vi "Main.vi"(11 "Module Admin":refnum<class "Delacor_lib_QMH_Module Admin.lvclass">) -> ()   [LabVIEW 2024, in "ControllerUI.lvlib"]
doc: "This template is based off of the Queued Message Handler design pattern and the Queued Message Handler project template that ships with LabVIEW.\n\nThe main difference is that the queue is private to this module and communication between modules is performed via Broadcast and Request events.\n\nRequest events are wrapped in public API methods and are handled in the Event Handling Loop (EHL) of this VI. Any module can register for Broadcast events sent by this module. The EHL generates messages based on user interface actions.\n\nThe Message Handling Loop (MHL) processes messages generated by the EHL, or by other messages. The messages are string values, so new messages can be added easily to the Message Cases case structure in the MHL. Each message cluster can also provide an optional value for Message Data, which is a variant that can be converted to whatever message-specific data is required.\n_____\nBased on DQMH Dev Tools: Project Template 7.1.0.1503."
uses:
  ControllerUI.lvlib
  <vilib>/Delacor/Delacor QMH/Libraries/Module Admin_class/Delacor_lib_QMH_Module Admin.lvclass
  Module Data--cluster.ctl
  <vilib>/Utility/miscctls.llb/LVFontTypeDef.ctl
  Stop Argument--cluster.ctl
  <vilib>/Delacor/Delacor QMH/Libraries/Message Queue_class/Delacor_lib_QMH_Message Queue.lvclass/Delacor_lib_QMH_Message Queue.ctl
  <vilib>/Delacor/Delacor QMH/Libraries/Module Admin_class/Delacor_lib_QMH_Module Admin.lvclass/Delacor_lib_QMH_Module Admin.ctl
  <vilib>/Delacor/Delacor QMH/Libraries/Message Queue_class/Delacor_lib_QMH_Enqueue Message (Single).vi
  <vilib>/Delacor/Delacor QMH/Libraries/Module Admin_class/Delacor_lib_QMH_Get External Launch.vi
  <vilib>/Delacor/Delacor QMH/Libraries/Message Queue_class/Delacor_lib_QMH_Message Queue.lvclass
  MoneyControl/MoneyControl.lvlib
  ProductControl/ProductControl.lvlib
  <vilib>/PantherLAB/Message Module/Libraries/Message/PantherLAB_lib_Message.lvlib
panel:
  out "error out":errorcluster
  out "Status":string
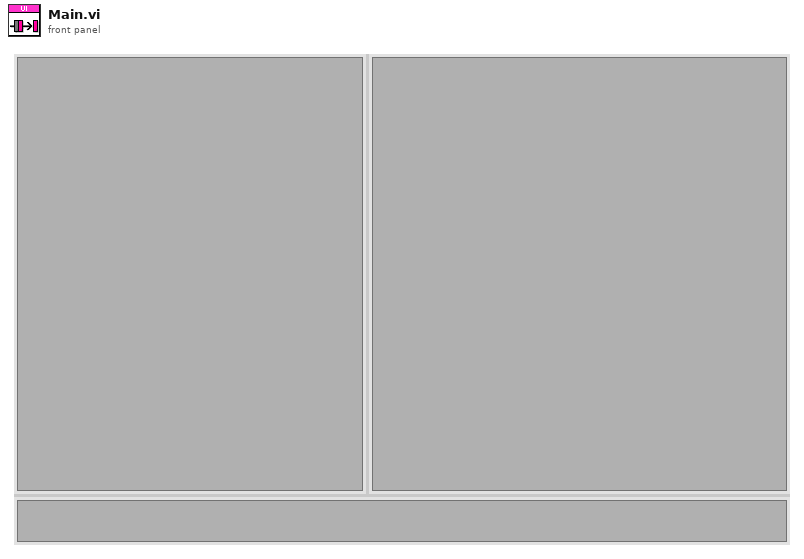
[diagram p1: front panel]
types:
  T1 = typedef "ControllerUI.lvlib/Request Events--cluster.ctl" = cluster{"Stop Module":refnum<user-event>, "Show Panel":refnum<user-event>, "Hide Panel":refnum<user-event>, "Get Module Execution Status":refnum<user-event>, "Show Diagram":refnum<user-event>}
  T2 = typedef "PantherLAB_lib_Message.lvlib/Broadcast Events--cluster.ctl" = cluster{"Module Did Init":refnum<user-event>, "Status Updated":refnum<user-event>, "Error Reported":refnum<user-event>, "Module Did Stop":refnum<user-event>, "Update Module Execution Status":refnum<user-event>}
  T3 = typedef "MoneyControl.lvlib/Broadcast Events--cluster.ctl" = cluster{"Module Did Init":refnum<user-event>, "Status Updated":refnum<user-event>, "Error Reported":refnum<user-event>, "Module Did Stop":refnum<user-event>, "Update Module Execution Status":refnum<user-event>, "Credito Actualizado":refnum<user-event>}
  T4 = typedef "ProductControl.lvlib/Broadcast Events--cluster.ctl" = cluster{"Module Did Init":refnum<user-event>, "Status Updated":refnum<user-event>, "Error Reported":refnum<user-event>, "Module Did Stop":refnum<user-event>, "Update Module Execution Status":refnum<user-event>, "Seleccion Producto Actualizada":refnum<user-event>}
  T5 = typedef "ControllerUI.lvlib/Module Data--cluster.ctl" = cluster{"Status":string}
  T6 = typedef "LVFontTypeDef.ctl" = cluster{"Font Name":string, "Size":u16, "Bold":bool, "Italic":bool, "Underline":bool, "Strikeout":bool, "Color":u32}
  T7 = enum32{"invalid lock state", "Not Locked", "Locked (No Password)", "Password-protected"}
  T8 = typedef "ControllerUI.lvlib/Stop Argument--cluster.ctl" = cluster{"Origin":string, "Exit via Stop Module Req?":bool, "Wait for Module to stop?":bool}
  T9 = enum32{"Invalid", "Standard", "Closed", "Hidden", "Minimized", "Maximized"}
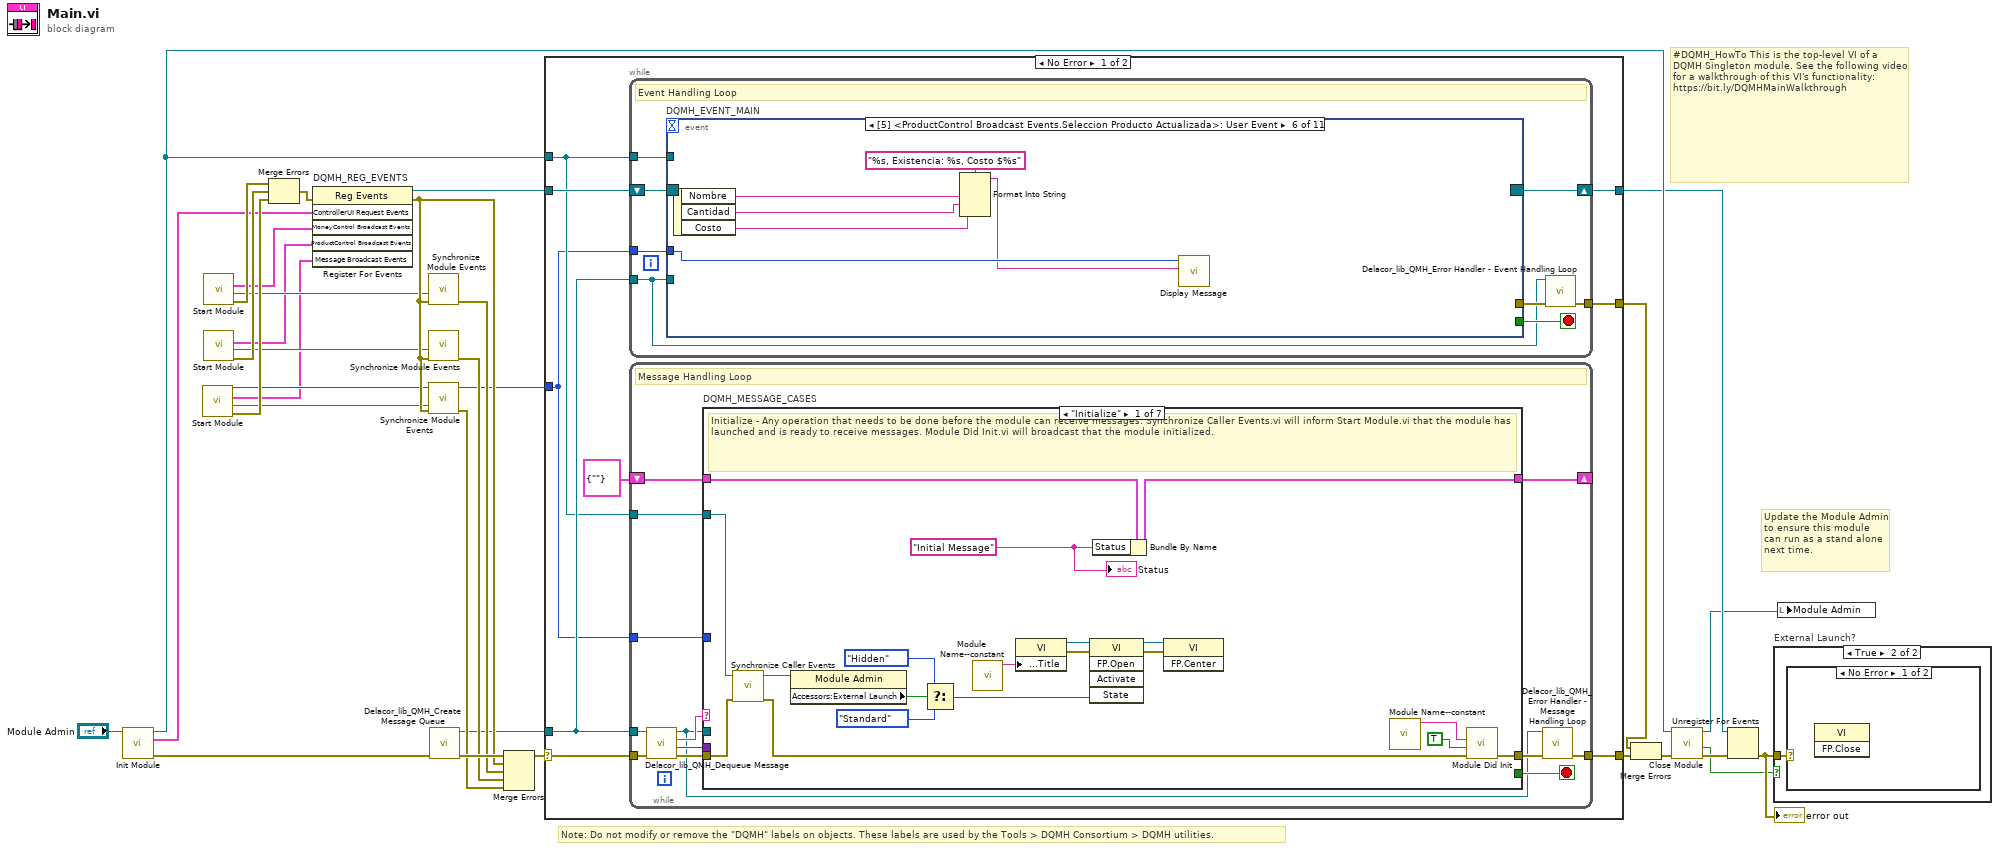
[diagram p0: block diagram]
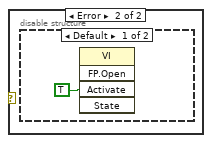
[diagram p3: hidden frame]
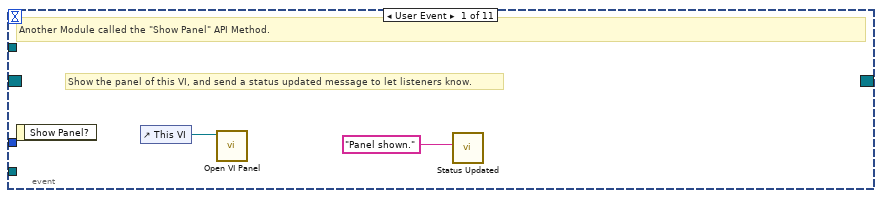
[diagram p5: hidden frame]
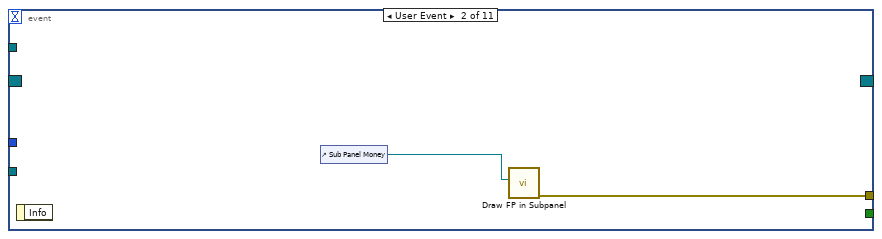
[diagram p6: hidden frame]
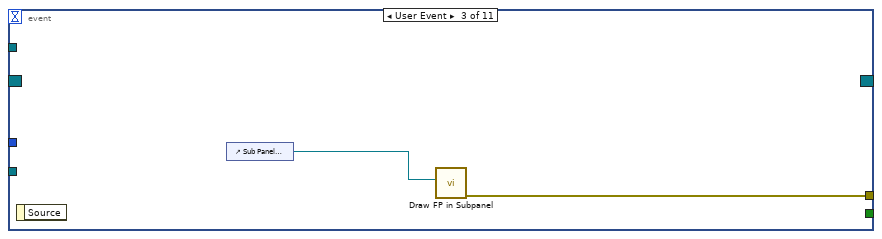
[diagram p7: hidden frame]
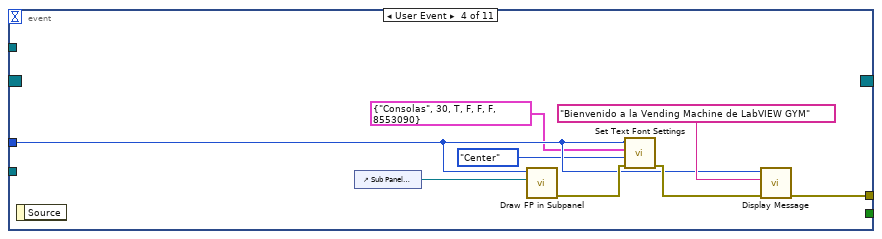
[diagram p8: hidden frame]
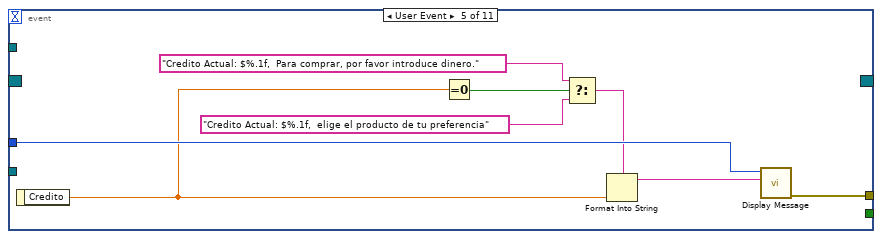
[diagram p9: hidden frame]
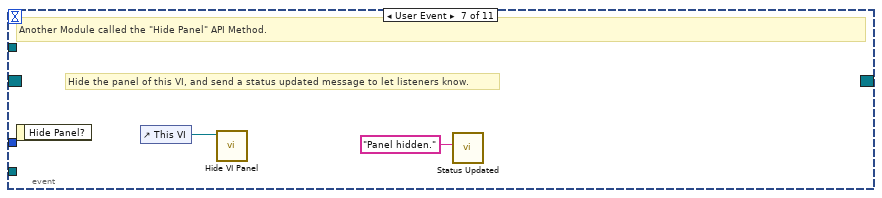
[diagram p10: hidden frame]
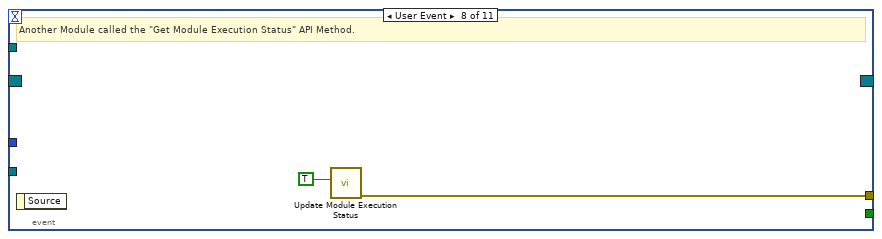
[diagram p11: hidden frame]
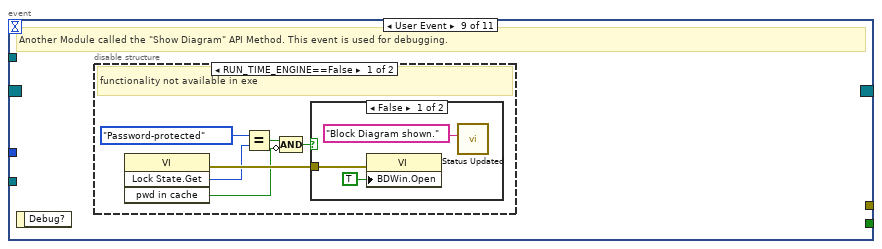
[diagram p12: hidden frame]
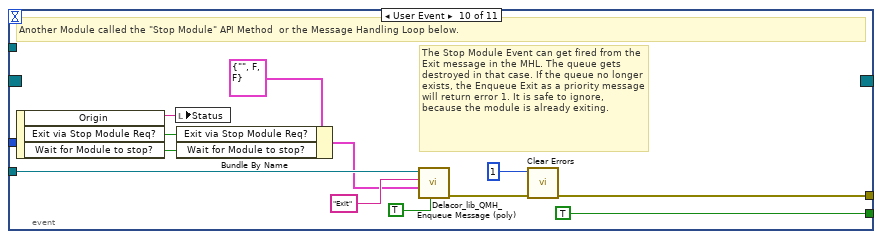
[diagram p15: hidden frame]
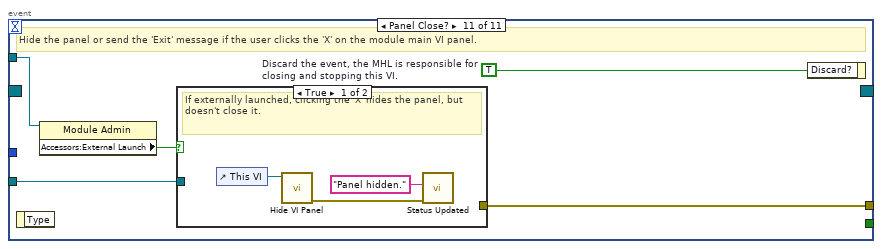
[diagram p16: hidden frame]
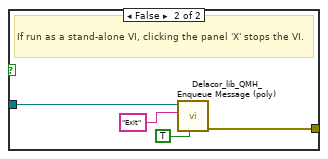
[diagram p17: hidden frame]
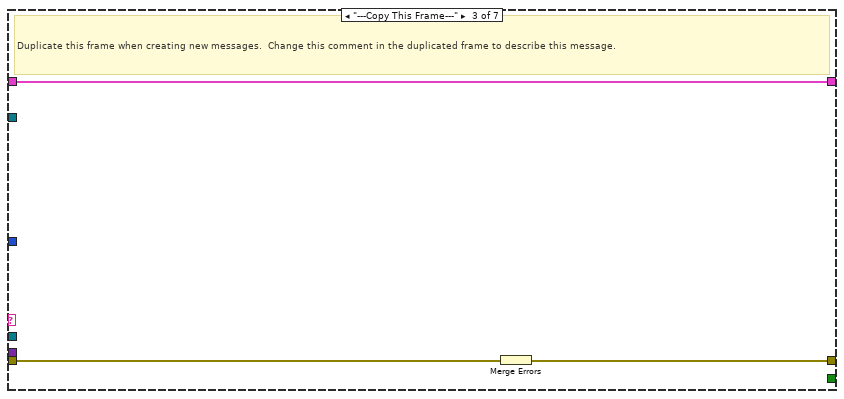
[diagram p19: hidden frame]
diagram:
  # "#DQMH_HowTo This is the top-level VI of a DQMH Singleton module. See the following video for a walkthrough of this VI's functionality: https://bit.ly/DQMHMainWalkthrough"
  # "Note: Do not modify or remove the \"DQMH\" labels on objects. These labels are used by the Tools > DQMH Consortium > DQMH utilities."
  # "Update the Module Admin to ensure this module can run as a stand alone next time."
  n1 = call "Init Module.vi"("Singleton Module Admin in"="Module Admin") -> ("error out"=w31:errorcluster, "ControllerUI Request Events"=w13:T1, "Singleton Module Admin out"=w16:refnum<class "Delacor_lib_QMH_Module Admin.lvclass">)  [unwired: 8 in]
  n2 = call <vilib>:"Start Module.vi"() -> ("error out"=w18:errorcluster, "Wait for Event Sync?"=w4:bool, "Message Broadcast Events"=w2:T2, "Module ID"=w3:i32)  [unwired: 7 in, 1 out]
  n3 = call <vilib>:"Start Module.vi"() -> ("error out"=w23:errorcluster, "Wait for Event Sync?"=w7:bool, "MoneyControl Broadcast Events"=w8:T3)  [unwired: 7 in, 2 out]
  n4 = call <vilib>:"Start Module.vi"() -> ("error out"=w22:errorcluster, "Wait for Event Sync?"=w5:bool, "ProductControl Broadcast Events"=w6:T4)  [unwired: 7 in, 2 out]
  n5 = Merge Errors(w23, w22, w18) -> (w24:errorcluster)
  n6 = register-events "DQMH_REG_EVENTS"(error in=w24, w13, w8, w6, w2) -> (reference out=w14:refnum<event-registration>, error out=w19:errorcluster)  [unwired: 1 in]
  n7 = call <vilib>:"Synchronize Module Events.vi"("error in"=w19, "Wait for Event Sync?"=w7) -> ("error out"=w21:errorcluster)  [unwired: 9 in]
  n8 = call <vilib>:"Synchronize Module Events.vi"("error in"=w19, "Wait for Event Sync?"=w5) -> ("error out"=w20:errorcluster)  [unwired: 9 in]
  n9 = call <vilib>:"Synchronize Module Events.vi"("error in"=w19, "Wait for Event Sync?"=w4, "Module ID in"=w3) -> ("error out"=w17:errorcluster, "Module ID out"=w1:i32)  [unwired: 7 in]
  n10 = call <vilib>:"Delacor_lib_QMH_Create Message Queue.vi"("error in"=w31) -> ("error out"=w26:errorcluster, "Message Queue"=w12:refnum<class "Delacor_lib_QMH_Message Queue.lvclass">)  [unwired: 9 in]
  n11 = Merge Errors(w26, w19, w21, w20, w17) -> (w25:errorcluster)
  n12 = case shown="No Error" w25 {
    selector: w25 -> [w39 w208]
    tunnel: [w41 w207] -> w32
    tunnel: [w38 w206] -> w15
    tunnel: w14 -> [w36 w206]
    tunnel: w12 -> [w35 w202]
    tunnel: [w40 _] -> w29
    tunnel: w16 -> [w34 w203]
    tunnel: w1 -> [w33 w201]
    frame No Error {
      n13 = while {
        tunnel: w35 -> [w43]
        shift-right: [w46] -> w38
        shift-left: w36 -> [w47]
        tunnel: [w48] -> w40
        tunnel: w34 -> [w44]
        tunnel: w33 -> [w42]
        stop <- w45 stop-if-true
        # "Event Handling Loop"
        n14 = event "DQMH_EVENT_MAIN" shown="[5] <ProductControl Broadcast Events.Seleccion Producto Actualizada>: User Event" {
          selector: w47 -> [_ _ _ _ _ _ _ _ _ _ _]
          dyn-events: [_ _ _ _ _ _ _ _ _ _ _] -> w46
          timeout: _ -> [_ _ _ _ _ _ _ _ _ _ _]
          tunnel: [_ _ _ _ _ _ _ _ _ TRUE ("Discard?") _] -> w45
          tunnel: w43 -> [_ _ _ _ _ _ _ _ _ w98 w105]
          tunnel: [_ w53 w55 w63 w71 _ _ w81 _ w101 w107] -> w49
          tunnel: w44 -> [_ _ _ _ _ _ _ _ _ _ w104]
          tunnel: w42 -> [_ _ _ w58 w70 w77 _ _ _ _ _]
          event User Event {
            # "Show the panel of this VI, and send a status updated message to let listeners know."
            # "Another Module called the \"Show Panel\" API Method."
            n15 = event-data() -> ()  [unwired: 1 in, 1 out]
            n16 = control-ref of="This VI"() -> (w51:refnum<vi>)
            n17 = call "Open VI Panel.vi"("VI"=w51) -> ()  [unwired: 10 in, 1 out]
            n18 = call "Status Updated.vi"("Status"="Panel shown." ("format string")) -> ()  [unwired: 10 in, 1 out]
          }
          event User Event {
            n19 = event-data() -> ()  [unwired: 1 in, 1 out]
            n20 = control-ref of="Sub Panel Money"() -> (w52:refnum<vi>)
            n21 = call <vilib>:"Draw FP in Subpanel.vi"("Sub Panel"=w52) -> ("error out"=w53:errorcluster)  [unwired: 10 in]
          }
          event User Event {
            n22 = event-data() -> ()  [unwired: 1 in, 1 out]
            n23 = control-ref of="Sub Panel Product"() -> (w54:refnum<vi>)
            n24 = call <vilib>:"Draw FP in Subpanel.vi"("Sub Panel"=w54) -> ("error out"=w55:errorcluster)  [unwired: 10 in]
          }
          event User Event {
            n25 = event-data() -> ()  [unwired: 1 in, 1 out]
            n26 = control-ref of="Sub Panel Mensajes"() -> (w60:refnum<vi>)
            n27 = call <vilib>:"Draw FP in Subpanel.vi"("Sub Panel"=w60, "Module ID"=w58) -> ("error out"=w62:errorcluster)  [unwired: 9 in]
            n28 = call <vilib>:"Set Text Font Settings.vi"("error in"=w62, "Text.Justification"=enum16{"Left", "Center", "Right"}."Center", "Font"=T6 {"Font Name"="Consolas", "Size"=30, "Bold"=TRUE, "Italic"=FALSE, "Underline"=FALSE, "Strikeout"=FALSE, "Color"=8553090}, "Module ID"=w58) -> ("error out"=w61:errorcluster)  [unwired: 7 in]
            n29 = call <vilib>:"Display Message.vi"("error in"=w61, "Message"="Bienvenido a la Vending Machine de LabVIEW GYM", "Module ID"=w58) -> ("error out"=w63:errorcluster)  [unwired: 8 in]
          }
          event User Event {
            n30 = event-data() -> ("Credito"=w68:dbl)  [unwired: 1 in]
            n31 = Equal To 0?(x=w68) -> (x = 0?=w67:bool)
            n32 = Select(t="Credito Actual: $%.1f,  Para comprar, por favor introduce dinero." ("format string"), s=w67, f="Credito Actual: $%.1f,  elige el producto de tu preferencia" ("format string")) -> (s? t:f=w65:string)
            n33 = Format Into String(format string=w65, w68) -> (resulting string=w69:string)  [unwired: 2 in, 1 out]
            n34 = call <vilib>:"Display Message.vi"("Message"=w69, "Module ID"=w70) -> ("error out"=w71:errorcluster)  [unwired: 9 in]
          }
          event User Event {
            n35 = event-data() -> ("Nombre"=w76:string, "Cantidad"=w75:string, "Costo"=w74:string)  [unwired: 1 in]
            n36 = Format Into String(format string="%s, Existencia: %s, Costo $%s", w76, w75, w74) -> (resulting string=w73:string)  [unwired: 2 in, 1 out]
            n37 = call <vilib>:"Display Message.vi"("Message"=w73, "Module ID"=w77) -> ()  [unwired: 9 in, 1 out]
          }
          event User Event {
            # "Hide the panel of this VI, and send a status updated message to let listeners know."
            # "Another Module called the \"Hide Panel\" API Method."
            n38 = event-data() -> ()  [unwired: 1 in, 1 out]
            n39 = control-ref of="This VI"() -> (w79:refnum<vi>)
            n40 = call "Hide VI Panel.vi"("VI"=w79) -> ()  [unwired: 10 in, 1 out]
            n41 = call "Status Updated.vi"("Status"="Panel hidden." ("format string")) -> ()  [unwired: 10 in, 1 out]
          }
          event User Event {
            # "Another Module called the \"Get Module Execution Status\" API Method."
            n42 = event-data() -> ()  [unwired: 1 in, 1 out]
            n43 = call "Update Module Execution Status.vi"("Running?"=TRUE) -> ("error out"=w81:errorcluster)  [unwired: 10 in]
          }
          event User Event {
            # "Another Module called the \"Show Diagram\" API Method. This event is used for debugging."
            n44 = event-data() -> ()  [unwired: 1 in, 1 out]
            n45 = disable-structure shown="RUN_TIME_ENGINE==False" {
              frame condition #0 (active) {
                # "functionality not available in exe"
                n46 = invoke on="Invoke Node" class="VI" method="Lock State.Get"() -> (error out=w87:errorcluster, "Get Lock State"=w86:T7, "pwd in cache"=w83:bool)  [unwired: 4 in, 1 out]
                n47 = Equal?(x=T7."Password-protected", y=w86) -> (x = y?=w84:bool)
                n48 = Compound Arithmetic op=AND(w84, invert w83) -> (w82:bool)
                n49 = case shown="False" w82 {
                  tunnel: w87 -> [w90 _]
                  frame False {
                    n50 = property on="Property Node" class="VI"(error in=w90, "BDWin.Open"=TRUE ("Block Diagram Window:Open")) -> ()  [unwired: 1 in, 2 out]
                    n51 = call "Status Updated.vi"("Status"="Block Diagram shown." ("format string")) -> ()  [unwired: 10 in, 1 out]
                  }
                  frame True {
                    # "Password-protected VI, and the password is not in the cache. Do not show the diagram."
                  }
                }
              }
              frame condition #1 {
              }
            }
          }
          event User Event {
            # "The Stop Module Event can get fired from the Exit message in the MHL. The queue gets destroyed in that case. If the queue no longer exists, the Enqueue Exit as a priority message will return error 1. It is safe to ignore, because the module is already exiting."
            # "Another Module called the \"Stop Module\" API Method  or the Message Handling Loop below."
            n52 = event-data() -> ("Origin"=w97:string, "Exit via Stop Module Req?"=w93:bool, "Wait for Module to stop?"=w92:bool)  [unwired: 1 in]
            n53 = local write "Status"(w97) -> ()
            n54 = Bundle By Name(cluster=T8 {"Origin"="", "Exit via Stop Module Req?"=FALSE, "Wait for Module to stop?"=FALSE} ("Stop Argument"), "Exit via Stop Module Req?"=w93, "Wait for Module to stop?"=w92) -> (w91:T8)
            n55 = call-poly <vilib>:"Delacor_lib_QMH_Enqueue Message (poly).vi"("Priority Message? (F)"=TRUE, "Message Data"=w91, "Message"="Exit", "Message Queue in"=w98) -> ("error out"=w102:errorcluster)  [unwired: 6 in, 1 out]
            n56 = call <vilib>:"Clear Errors.vi"("error in (no error)"=w102, "specific error code to clear (0: all)"=1) -> ("error out"=w101:errorcluster)  [unwired: 4 in, 1 out]
          }
          event Panel Close? {
            w106 = TRUE  # Discard the event, the MHL is responsible for closing and stopping this VI.
            # "Hide the panel or send the 'Exit' message if the user clicks the 'X' on the module main VI panel."
            n57 = event-data() -> ()  [unwired: 1 in, 1 out]
            n58 = property on="Property Node" class="Module Admin"(reference=w104) -> ("Accessors:External Launch"=w103:bool)  [unwired: 1 in, 2 out]
            n59 = case shown="True" w103 {
              tunnel: w105 -> [_ w113]
              tunnel: [_ w114] -> w107
              frame True {
                # "If externally launched, clicking the 'X' hides the panel, but doesn't close it."
                n60 = control-ref of="This VI"() -> (w109:refnum<vi>)
                n61 = call "Hide VI Panel.vi"("VI"=w109) -> ("error out"=w110:errorcluster)  [unwired: 10 in]
                n62 = call "Status Updated.vi"("error in"=w110, "Status"="Panel hidden." ("format string")) -> ()  [unwired: 9 in, 1 out]
              }
              frame False {
                # "If run as a stand-alone VI, clicking the panel 'X' stops the VI."
                n63 = call-poly <vilib>:"Delacor_lib_QMH_Enqueue Message (poly).vi"("Priority Message? (F)"=TRUE, "Message"="Exit", "Message Queue in"=w113) -> ("error out"=w114:errorcluster)  [unwired: 7 in, 1 out]
              }
            }
            n64 = event-data ("Event Filter Node")("Discard?"=w106) -> ()  [unwired: 1 in, 1 out]
          }
        }
        n65 = call-dynamic "Delacor_lib_QMH_Error Handler - Event Handling Loop.vi"("error in"=w49, "Message Queue in"=w43) -> ("dup error in"=w48:errorcluster)  [unwired: 8 in, 1 out]
      }
      n66 = while {
        tunnel: w35 -> [w116]
        shift-right: [w122] -> _
        shift-left: T5 {"Status"=""} ("Data Cluster") -> [w123]
        tunnel: w39 -> [w127]
        tunnel: [w125] -> w41
        tunnel: w34 -> [w118]
        tunnel: w33 -> [w115]
        stop <- w121 stop-if-true
        # "Message Handling Loop"
        n67 = call-dynamic "Delacor_lib_QMH_Dequeue Message.vi"("error in"=w127, "Message Queue in"=w116) -> ("error out"=w126:errorcluster, "Message Data"=w119:variant, "Message"=w120:string, "Message Queue out"=w117:refnum<class "Delacor_lib_QMH_Message Queue.lvclass">)  [unwired: 6 in]
        n68 = case "DQMH_MESSAGE_CASES" shown="\"Initialize\"" w120 {
          selector: w120 -> [_ _ _ _ _ _ w195]
          tunnel: w117 -> [_ _ _ _ w156 w183 _]
          tunnel: w126 -> [w144 w148 w151 w153 w164 w189 w198]
          tunnel: [w142 w148 w150 w153 w160 w184 w199] -> w124
          tunnel: w123 -> [w133 w147 w149 w152 w158 w182 w196]
          tunnel: [w132 w147 w149 w152 w158 w182 w196] -> w122
          tunnel: [_ _ _ _ _ w181 _] -> w121
          tunnel: w119 -> [_ _ _ _ w157 w180 _]
          tunnel: w118 -> [w134 _ _ _ w155 w175 _]
          tunnel: w115 -> [_ _ _ _ _ w174 _]
          frame "Initialize" {
            w128 = "Initial Message" ("Initial Message")
            # "Initialize - Any operation that needs to be done before the module can receive messages. Synchronize Caller Events.vi will inform Start Module.vi that the module has launched and is ready to receive messages. Module Did Init.vi will broadcast that the module initialized."
            n69 = call "Synchronize Caller Events.vi"("error in"=w144, "Singleton Module Admin in"=w134) -> ("error out"=w143:errorcluster, "Singleton Module Admin out"=w129:refnum<class "Delacor_lib_QMH_Module Admin.lvclass">)  [unwired: 8 in]
            n70 = property on="Property Node" class="Module Admin"(reference=w129) -> ("Accessors:External Launch"=w138:bool)  [unwired: 1 in, 2 out]
            n71 = Select(t=T9."Hidden" ("State"), s=w138, f=T9."Standard" ("State")) -> (s? t:f=w135:T9)
            n72 = call "Module Name--constant.vi"() -> ("Module Name"=w141:string)  [unwired: 11 in]
            n73 = property on="Property Node" class="VI"("Front Panel.Title"=w141) -> (reference out=w140:refnum<vi>, error out=w146:errorcluster)  [unwired: 2 in]
            n74 = invoke on="Invoke Node" class="VI" method="FP.Open"(reference=w140, error in=w146, "State"=w135) -> (reference out=w139:refnum<vi>, error out=w145:errorcluster)  [unwired: 2 in, 3 out]
            n75 = Bundle By Name(cluster=w133, "Status"=w128) -> (w132:T5)
            n76 = invoke on="Invoke Node" class="VI" method="FP.Center"(reference=w139, error in=w145) -> ()  [unwired: 1 in, 3 out]
            n77 = call "Module Name--constant.vi"() -> ("Module Name"=w130:string)  [unwired: 11 in]
            n78 = call "Module Did Init.vi"("error in"=w143, "Initialized?"=TRUE, "Origin"=w130) -> ("error out"=w142:errorcluster)  [unwired: 8 in]
            "Status" <- w128
          }
          frame "---Module Specific---" {
            # "Separator -- The following cases handle messages specific to this Module."
          }
          frame "---Copy This Frame---" {
            # "Duplicate this frame when creating new messages.  Change this comment in the duplicated frame to describe this message."
            n79 = Merge Errors(w151) -> (w150:errorcluster)
          }
          frame "---Exit and Error Handling---" {
            # "Separator - The following cases handle errors and exit messages."
          }
          frame "Error" {
            # "#DQMH_CodeRecommended - If the module is running in standalone mode (External Launch = FALSE), this code will pop up an error dialog and call the 'Exit' message if an error occurs. Add more fine-grained error management here."
            # "Error - Check the error message data and respond accordingly. This message is sent by the \"Error Handler\" VIs at the end of each loop in this application."
            n80 = property on="Property Node" class="Module Admin"(reference=w155) -> ("Accessors:External Launch"=w154:bool)  [unwired: 1 in, 2 out]
            n81 = Variant To Data(error in=w164, type=errorcluster {"status"=FALSE, "code"=0, "source"=""} ("error constant"), Variant=w157) -> (data=w159:errorcluster, error out=w162:errorcluster)
            n82 = local write "error out"(w159) -> ()
            n83 = call "Error Reported.vi"("Error"=w159) -> ()  [unwired: 10 in, 1 out]
            n84 = case shown="False" w154 {
              tunnel: [w169 _] -> w161
              tunnel: w156 -> [w167 _]
              tunnel: w159 -> [w168 _]
              frame False {
                n85 = disable-structure shown="Default" {
                  disable-tunnel: w168 -> [w170 _]
                  frame condition #0 (active) {
                    # "If the module is running standalone, then pop up an error dialog and call the \"Exit\" message."
                    n86 = call <vilib>:"Simple Error Handler.vi"("error in (no error)"=w170) -> ()  [unwired: 4 in, 5 out]
                  }
                  frame condition #1 {
                    # "To prevent the Simple Error Handler VI from being loaded (e.g. when deploying to a Real-Time target), add the Conditional Disable Symbol \"DQMH_Disable_SEH\" to your project and set it to TRUE."
                  }
                }
                n87 = call-poly <vilib>:"Delacor_lib_QMH_Enqueue Message (poly).vi"("Priority Message? (F)"=TRUE, "Message"="Exit", "Message Queue in"=w167) -> ("error out"=w169:errorcluster)  [unwired: 7 in, 1 out]
              }
              frame True {
                # "If the module was launched externally, calling the Error Reported broadcast VI is the only action performed by the \"Error\" message. The module's caller can then process the error appropriately."
              }
            }
            n88 = Merge Errors(w162, w161) -> (w160:errorcluster)
          }
          frame "Exit" {
            w179 = 91  # 91: not all Exit messages will have an argument
            w181 = TRUE  # Stop the VI
            # "Release the message queue reference"
            # "Exit - Exit the application."
            n89 = Variant To Data(error in=w189, type=T8 {"Origin"="", "Exit via Stop Module Req?"=FALSE, "Wait for Module to stop?"=FALSE} ("Stop Argument"), Variant=w180) -> (data=w177:T8, error out=w186:errorcluster)
            n90 = call <vilib>:"Clear Errors.vi"("error in (no error)"=w186, "specific error code to clear (0: all)"=w179) -> ("error out"=w188:errorcluster)  [unwired: 4 in, 1 out]
            n91 = control-ref of="This VI"() -> (w176:refnum<vi>)
            n92 = call-dynamic "Delacor_lib_QMH_Release Message Queue.vi"("error in"=w188, "Message Queue"=w183) -> ("error out"=w187:errorcluster)  [unwired: 9 in]
            n93 = call "Handle Exit.vi"("Stop Argument"=w177, "Admin in"=w175, "VI reference"=w176) -> ("error out"=w185:errorcluster)  [unwired: 7 in, 1 out]
            n94 = Merge Errors(w187, w185) -> (w184:errorcluster)
            n95 = call "Error Reported.vi"("Error"=w184) -> ()  [unwired: 10 in, 1 out]
            n96 = call "Module Name--constant.vi"() -> ("Module Name"=w173:string)  [unwired: 11 in]
            n97 = Format Into String(format string="%s Sent Stop.", w173) -> (resulting string=w172:string)  [unwired: 2 in, 1 out]
            n98 = call <vilib>:"Stop Module.vi"("Origin"=w172) -> ()  [unwired: 10 in, 1 out]
            n99 = call <vilib>:"Stop Module.vi"("Origin"=w172) -> ()  [unwired: 10 in, 1 out]
            n100 = call <vilib>:"Stop Module.vi"("Origin"=w172, "Module ID"=w174) -> ()  [unwired: 9 in, 1 out]
          }
          frame Default {
            # "'Default' case only runs if there is a message that isn't defined in any of the other cases.  Output a programming error."
            n101 = call "Module Name--constant.vi"() -> ("Module Name"=w194:string)  [unwired: 11 in]
            n102 = Format Into String(format string="The invalid message string \"%s\" was received in the Message Handling Loop for module \"%s\".", w195, w194) -> (resulting string=w190:string)  [unwired: 2 in, 1 out]
            n103 = call <vilib>:"Error Cluster From Error Code.vi"("show call chain? (False)"=TRUE, "error message (\"\")"=w190, "error code (0)"=1) -> ("error out"=w197:errorcluster)  [unwired: 6 in]
            n104 = Merge Errors(w198, w197) -> (w199:errorcluster)
          }
        }
        n105 = call-dynamic "Delacor_lib_QMH_Error Handler - Message Handling Loop.vi"("error in"=w124, "Message Queue in"=w117) -> ("dup error in"=w125:errorcluster)  [unwired: 8 in, 1 out]
      }
    }
    frame Error {
      # "Synchronize Caller Events.vi will inform Start Module.vi that the module has launched and will let the code calling Start Module.vi register for broadcasts and would permit the caller receive the broadcast that an error occurred at launch time."
      n106 = call-dynamic "Delacor_lib_QMH_Release Message Queue.vi"("error in"=w208, "Message Queue"=w202) -> ("error out"=w207:errorcluster)  [unwired: 9 in]
      n107 = call "Synchronize Caller Events.vi"("Singleton Module Admin in"=w203) -> ("error out"=w209:errorcluster)  [unwired: 9 in, 1 out]
      n108 = call "Module Name--constant.vi"() -> ("Module Name"=w205:string)  [unwired: 11 in]
      n109 = Format Into String(format string="An error occurred during initialization. %s is no longer running.", w205) -> (resulting string=w200:string)  [unwired: 2 in, 1 out]
      n110 = Merge Errors(w207, w209) -> (w210:errorcluster)
      n111 = call "Error Reported.vi"("Additional Information"=w200, "Error"=w210) -> ()  [unwired: 9 in, 1 out]
      n112 = call <vilib>:"Stop Module.vi"("Origin"=w200) -> ()  [unwired: 10 in, 1 out]
      n113 = call <vilib>:"Stop Module.vi"("Origin"=w200) -> ()  [unwired: 10 in, 1 out]
      n114 = call <vilib>:"Stop Module.vi"("Origin"=w200, "Module ID"=w201) -> ()  [unwired: 9 in, 1 out]
    }
  }
  n115 = Merge Errors(w29, w32) -> (w28:errorcluster)
  n116 = call "Close Module.vi"("error in"=w28, "Module Admin in"=w16) -> ("error out"=w30:errorcluster, "External Launch"=w9:bool, "Module Admin out"=w10:refnum<class "Delacor_lib_QMH_Module Admin.lvclass">)  [unwired: 7 in]
  n117 = Unregister For Events(event registration refnum=w15, error in=w30) -> (error out=w27:errorcluster)
  "error out" <- w27
  n118 = case "External Launch?" shown="True" w9 {
    tunnel: w27 -> [_ w211]
    frame False {
    }
    frame True {
      n119 = case shown="No Error" w211 {
        frame No Error {
          n120 = invoke on="Invoke Node" class="VI" method="FP.Close"() -> ()  [unwired: 3 in, 3 out]
        }
        frame Error {
          n121 = disable-structure shown="Default" {
            frame condition #0 (active) {
              n122 = invoke class="VI" method="FP.Open"("Activate"=TRUE ("Activate?")) -> ()  [unwired: 4 in, 5 out]
            }
            frame condition #1 {
              # "Don't show panel on error if running inside a built EXE."
            }
          }
        }
      }
    }
  }
  n123 = local write "Module Admin"(w10) -> ()
